vi "PostMessage Master.vi"(8 "error in":errorcluster caption="error in (no error)" {"code" format="%d\n%x"}, 10 "Function":T2(ring), 11 "window refnum":T1) -> (0 "error out":errorcluster {"code" format="%d\n%x"}, 3 "window refnum out":T1)   [LabVIEW 2020, in "MacroAssert.lvlib" / "Win Util New.lvlib"]
doc: "This VI acts as a \"Master\" for various VIs that use the LVPostMessage function in the LVWUTIL.DLL library. This is basically just the PostMessage API function with a WM_SYSCOMMAND message, but also does some additional checking for the existance of the targeted window."
uses:
  Win Util New.lvlib
  Window Refnum.ctl
  user32.dll
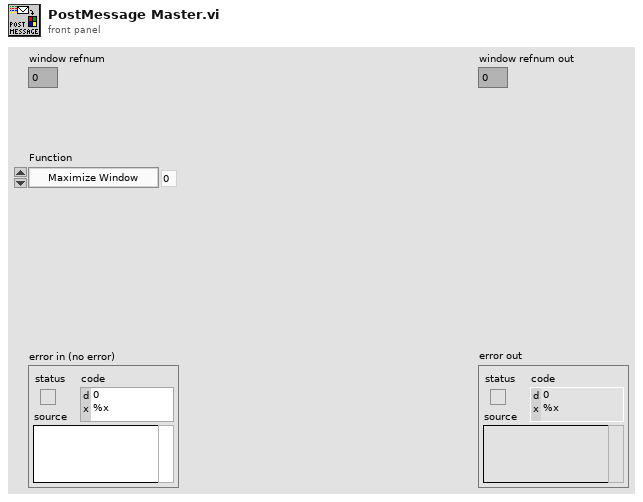
[diagram p1: front panel]
types:
  T1 = typedef "MacroAssert.lvlib/Win Util New.lvlib/Window Refnum.ctl" = u64
  T2 = enum8{"Maximize Window", "Minimize Window", "Show Task List", "Start Screen Saver", "Quit Application"}
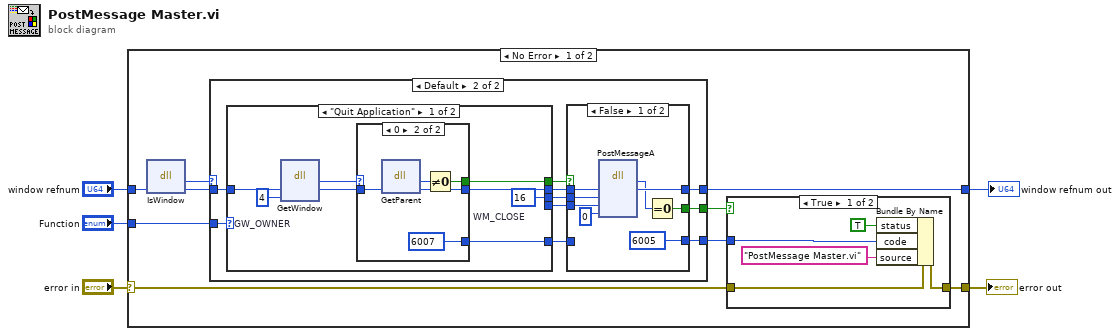
[diagram p0: block diagram]
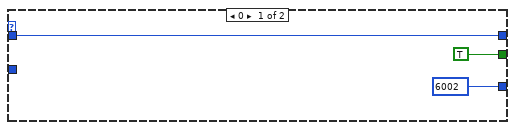
[diagram p2: hidden frame]
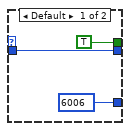
[diagram p4: hidden frame]
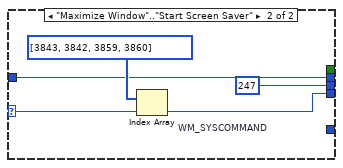
[diagram p5: hidden frame]
diagram:
  n1 = case shown="No Error" "error in" {
    selector: "error in" -> [w12 w66]
    tunnel: [w14 w66] -> w5
    tunnel: "window refnum" -> [w8 w67]
    tunnel: [w13 w67] -> w2
    tunnel: "Function" -> [w6 _]
    frame No Error {
      n2 = dll-call lib="user32.dll" fn="IsWindow"("hWnd"=w8) -> ("IsWindow?"=w9:i32, "hWnd"=w7:u64)  [unwired: 3 in, 2 out]
      n3 = case shown="Default" w9 {
        tunnel: w7 -> [w17 w21]
        tunnel: [w17 w24] -> w13
        tunnel: [6002 w26] -> w11
        tunnel: [TRUE w25] -> w10
        tunnel: w6 -> [_ w27]
        frame 0 {
        }
        frame Default {
          n4 = case shown="\"Quit Application\"" w27 {
            selector: w27 -> [_ w58]
            tunnel: [w46 w57] -> w23
            tunnel: [_ w56] -> w22
            tunnel: [w43 w55] -> w20
            tunnel: w21 -> [w45 w55]
            tunnel: [w41 _] -> w19
            tunnel: [w40 _] -> w18
            frame "Quit Application" {
              w39 = u32 4  # GW_OWNER
              w46 = u32 16  # WM_CLOSE
              n5 = dll-call lib="user32.dll" fn="GetWindow"("hWnd"=w45, "uCmd"=w39) -> ("return type"=w42:u64, "hWnd"=w44:u64)  [unwired: 4 in, 2 out]
              n6 = case shown="0" w42 {
                tunnel: w44 -> [w49 w54]
                tunnel: [w49 w53] -> w43
                tunnel: [TRUE w51] -> w41
                tunnel: [6006 6007] -> w40
                frame Default {
                }
                frame 0 {
                  n7 = dll-call lib="user32.dll" fn="GetParent"("hWnd"=w54) -> ("return type"=w52:u64, "hWnd"=w53:u64)  [unwired: 3 in, 2 out]
                  n8 = Not Equal To 0?(x=w52) -> (x != 0?=w51:bool)
                }
              }
            }
            frame "Maximize Window".."Start Screen Saver" {
              w57 = u32 247  # WM_SYSCOMMAND
              n9 = Index Array(array=u64[] [3843, 3842, 3859, 3860], index=w58) -> (element=w56:u64)
            }
          }
          n10 = case shown="False" w19 {
            selector: w19 -> [_ w36]
            tunnel: [6005 w38] -> w26
            tunnel: [w34 w36] -> w25
            tunnel: [w33 w37] -> w24
            tunnel: w23 -> [w32 _]
            tunnel: w22 -> [w31 _]
            tunnel: w20 -> [w30 w37]
            tunnel: w18 -> [_ w38]
            frame False {
              n11 = dll-call lib="user32.dll" fn="PostMessageA" label="PostMessage"("hWnd"=w30, "Msg"=w32, "wParam"=w31, "lParam"=i64 0) -> ("error code"=w28:i32, "hWnd"=w33:u64)  [unwired: 6 in, 2 out]
              n12 = Equal To 0?(x=w28) -> (x = 0?=w34:bool)
            }
            frame True {
            }
          }
        }
      }
      n13 = case shown="True" w10 {
        tunnel: [w64 w65] -> w14
        tunnel: w12 -> [w63 w65]
        tunnel: w11 -> [w62 _]
        frame True {
          n14 = Bundle By Name(cluster=w63, "status"=TRUE, "code"=w62, "source"="PostMessage Master.vi") -> (w64:errorcluster)
        }
        frame False {
        }
      }
    }
    frame Error {
    }
  }
  "error out" <- w5
  "window refnum out" <- w2
